vi "Set Array of Points to Measure.vi"(8 "error in":errorcluster, 10 "array of points to measure":T1[](array[typedef]), 11 "eye scan in":refnum<class "niHighSpeedSerial N Point Eye Scan v1 Host.lvclass">) -> (0 "error out":errorcluster, 3 "eye scan out":refnum<class "niHighSpeedSerial N Point Eye Scan v1 Host.lvclass">)   [LabVIEW 2014, in "niHighSpeedSerial N Point Eye Scan v1 Host.lvclass"]
doc: "Sets the array of point offsets to measure.\n\n<B>Input Parameters</B>\n\n<B>error in</B> describes error conditions that occur before this node runs. This input provides standard 'error in' functionality.\n\n<B>array of points to measure</B> is the array of point offsets to measure using Eye Scan.\n\n<B>array of points to measure.horizontal offset</B> is the horizontal offset of the point to measure.\n\n<B>array of points to measure.vertical offset</B> is the vertical offset of the point to measure.\n\n<B>eye scan in</B> Takes in a reference to your session from the previous VI.\n\n<B>Output Parameters</B>\n\n<B>error out</B> contains error information. This output provides standard 'error out' functionality.\n\n<B>eye scan out</B> passes a reference to your session to the next VI."
uses:
  <instrlib>/niHighSpeedSerial/Eye Scan/v1/Host/Impl/N Point Eye Scan/niHighSpeedSerial N Point Eye Scan v1 Host.lvclass
  <instrlib>/niHighSpeedSerial/Eye Scan/v1/Host/Common/Public/Point Offsets.ctl
  <instrlib>/niHighSpeedSerial/Eye Scan/v1/Host/Impl/N Point Eye Scan/niHighSpeedSerial N Point Eye Scan v1 Host.lvclass/niHighSpeedSerial N Point Eye Scan v1 Host.ctl
  <vilib>/Utility/error.llb/Error Cluster From Error Code.vi
  <vilib>/ErrorRing/Error Ring.xnode
  <instrlib>/niHighSpeedSerial/Eye Scan/v1/Host/Eye Scan/niHighSpeedSerial Eye Scan v1 Host.lvclass
  <instrlib>/niHighSpeedSerial/Eye Scan/v1/Host/Common/niHighSpeedSerial Eye Scan Common v1 Host.lvlib
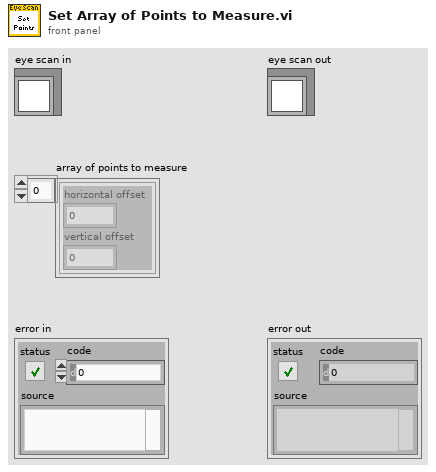
[diagram p1: front panel]
types:
  T1 = typedef "niHighSpeedSerial Eye Scan Common v1 Host.lvlib/Point Offsets.ctl" = cluster{"horizontal offset":i16, "vertical offset":i8}
  T2 = typedef "N Point Eye Scan v1 Host.lvclass/Private Data.ctl" = cluster{"array of points to measure":T1[], "n point eye scan point iterator":refnum<class "niHighSpeedSerial N Point Eye Scan Point Iterator v1 Host.lvclass">}
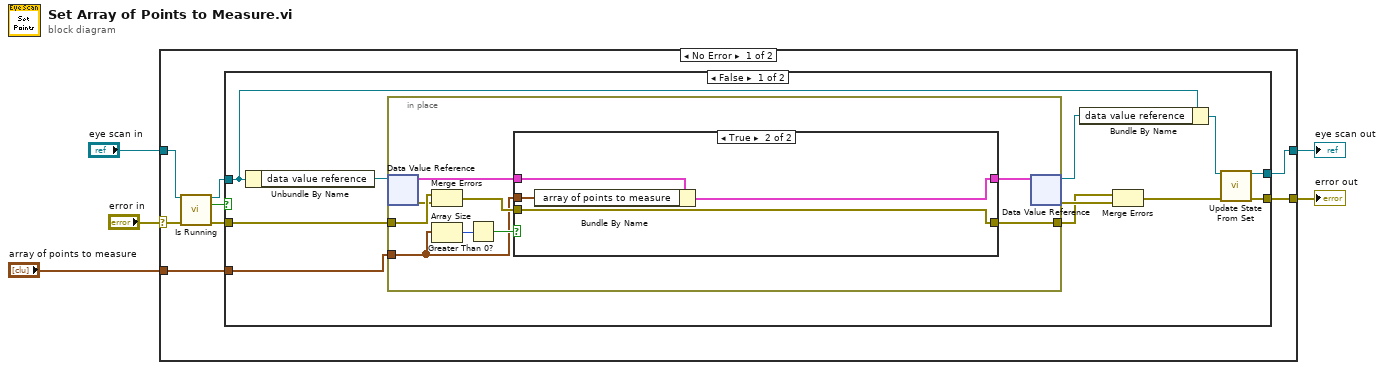
[diagram p0: block diagram]
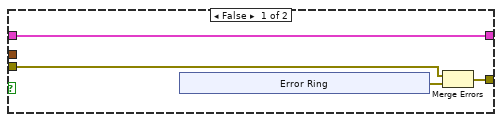
[diagram p2: hidden frame]
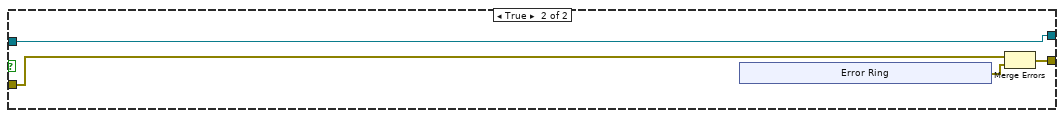
[diagram p3: hidden frame]
diagram:
  n1 = case shown="No Error" "error in" {
    selector: "error in" -> [w8 w55]
    tunnel: [w11 w55] -> w4
    tunnel: [w12 w54] -> w3
    tunnel: "eye scan in" -> [w10 w54]
    tunnel: "array of points to measure" -> [w13 _]
    frame No Error {
      n2 = call <instrlib>:"Is Running.vi"("eye scan in"=w10, "error in"=w8) -> ("eye scan out"=w9:refnum<class "niHighSpeedSerial N Point Eye Scan v1 Host.lvclass">, "is running?"=w6:bool, "error out"=w7:errorcluster)  [unwired: 11 in]
      n3 = case shown="False" w6 {
        tunnel: w13 -> [w20 _]
        tunnel: [w16 w46] -> w12
        tunnel: [w14 w47] -> w11
        tunnel: w9 -> [w19 w46]
        tunnel: w7 -> [w18 w48]
        frame False {
          n4 = Unbundle By Name(w19) -> ("data value reference"=w24:refnum<data-value>)
          n5 = in-place {
            in-place-border: w20 -> [w26]
            in-place-border: w18 -> [w33]
            in-place-border: [w28] -> w21
            n6 = in-place-dvr #1(w24) -> (w25:T2, w32:errorcluster)
            n7 = Merge Errors(w33, w32) -> (w29:errorcluster)
            n8 = Array Size(array=w26) -> (size(s)=w30:i32)
            n9 = Greater Than 0?(x=w30) -> (x > 0?=w31:bool)
            n10 = case shown="True" w31 {
              tunnel: [w37 w45] -> w28
              tunnel: w29 -> [w36 w45]
              tunnel: w25 -> [w35 w44]
              tunnel: [w35 w43] -> w27
              tunnel: w26 -> [_ w42]
              frame False {
                n11 = xnode "Error Ring"() -> ("error out"=w34:errorcluster)
                n12 = Merge Errors(w36, w34) -> (w37:errorcluster)
              }
              frame True {
                n13 = Bundle By Name(cluster=w44, "array of points to measure"=w42) -> (w43:T2)
              }
            }
            n14 = in-place-dvr #1(w27) -> (w23:refnum<data-value>, w22:errorcluster)
          }
          n15 = Bundle By Name(cluster=w19, "data value reference"=w23) -> (w17:refnum<class "niHighSpeedSerial N Point Eye Scan v1 Host.lvclass">)
          n16 = Merge Errors(w21, w22) -> (w15:errorcluster)
          n17 = call <instrlib>:"Update State From Set.vi"("eye scan in"=w17, "error in"=w15) -> ("eye scan out"=w16:refnum<class "niHighSpeedSerial N Point Eye Scan v1 Host.lvclass">, "error out"=w14:errorcluster)  [unwired: 12 in]
        }
        frame True {
          n18 = xnode "Error Ring"() -> ("error out"=w49:errorcluster)
          n19 = Merge Errors(w48, w49) -> (w47:errorcluster)
        }
      }
    }
    frame Error {
    }
  }
  "eye scan out" <- w3
  "error out" <- w4
